vi "reportTestStatus.vi"(7 "TaskRef":refnum<vi>, 8 "error in (no error)":errorcluster, 10 "TestResult":T1, 11 "pdbm_taskroute_feedback_event":refnum<user-event>) -> (0 "error out":errorcluster, 3 "pdbm_taskroute_feedback_event out":refnum<user-event>, 5 "TaskRef out":refnum<vi>)   [LabVIEW 2010, in "pdbm_tasks.lvlib"]
uses:
  pdbm_tasks.lvlib
  pdbm_test_route/UsrDefine/TaskFeedbackCmd.ctl
  UsrDefine/TestResult.ctl
  UsrDefine/TaskRequest.ctl
  pdbm_test_route/pdbm_task_route.lvlib
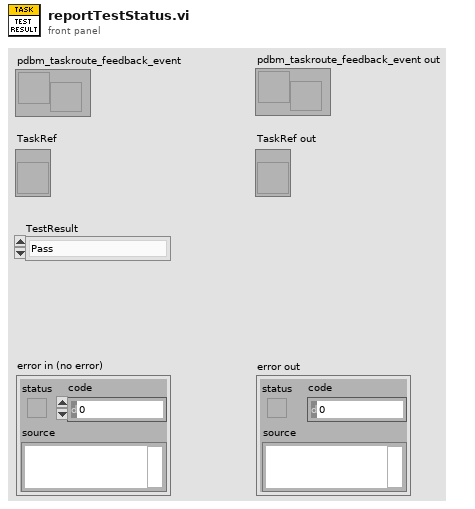
[diagram p1: front panel]
types:
  T1 = typedef "pdbm_tasks.lvlib/TestResult.ctl" = enum16{"Pass", "Fail", "Warning"}
  T2 = typedef "pdbm_tasks.lvlib/TaskRequest.ctl" = cluster{"Command":string, "Variant":variant}
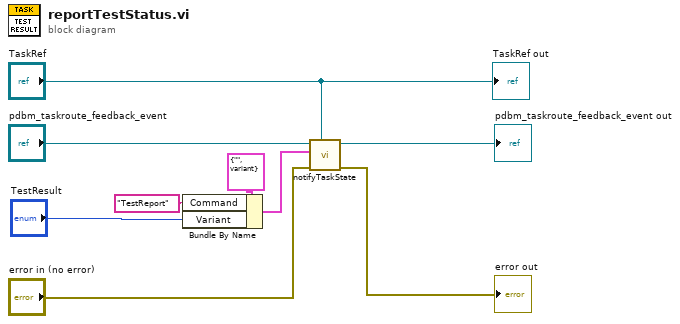
[diagram p0: block diagram]
diagram:
  n1 = Bundle By Name(cluster=T2 {"Command"="", "Variant"=variant} ("TaskRequest"), "Command"="TestReport", "Variant"="TestResult") -> (w7:T2)
  n2 = call "notifyTaskState.vi"("TaskRef"="TaskRef", "error in (no error)"="error in (no error)", "TaskRequest"=w7, "pdbm_taskroute_feedback_event"="pdbm_taskroute_feedback_event") -> ("error IO"=→"error out":errorcluster, "pdbm_taskroute_feedback_event out"=→"pdbm_taskroute_feedback_event out":refnum<user-event>)  [unwired: 6 in]
  "TaskRef out" <- "TaskRef"
